vi "PT100.vi"(1 "R":dbl=-0.05) -> (0 "T":dbl)   [LabVIEW 2009]
panel:
  out "output cluster":cluster{dbl[], dbl[]}
  out "XY Graph":cluster{dbl[], dbl[]}(graph)
  in  "t":dbl=-0.05
  out "Rout":dbl
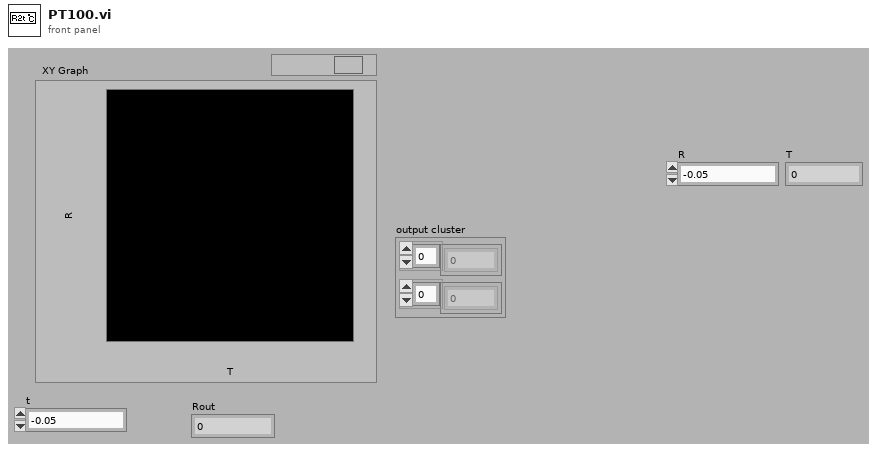
[diagram p1: front panel]
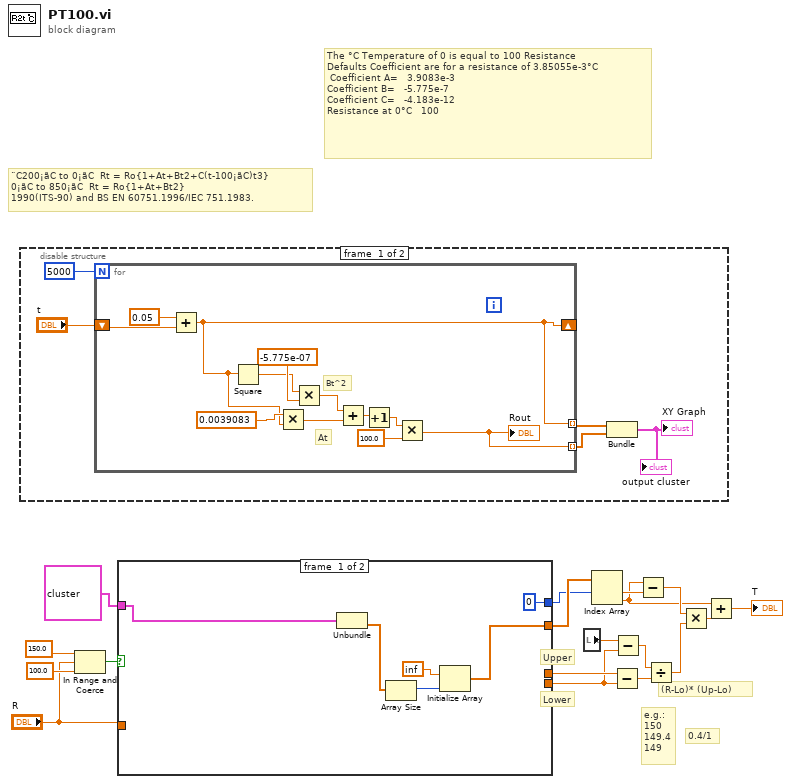
[diagram p0: block diagram]
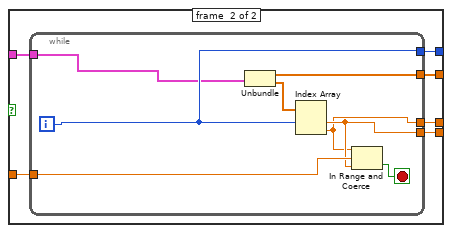
[diagram p3: hidden frame]
diagram:
  # "0.4/1"
  # "e.g.:\n150\n149.4\n149"
  # "(R-Lo)* (Up-Lo)"
  # "Lower"
  # "Upper"
  # "The °C Temperature of 0 is equal to 100 Resistance\nDefaults Coefficient are for a resistance of 3.85055e-3°C\n Coefficient A=   3.9083e-3 \nCoefficient B=   -5.775e-7 \nCoefficient C=   -4.183e-12 \nResistance at 0°C   100"
  # "¨C200¡ãC to 0¡ãC  Rt = Ro{1+At+Bt2+C(t-100¡ãC)t3} \n0¡ãC to 850¡ãC  Rt = Ro{1+At+Bt2} \n1990(ITS-90) and BS EN 60751.1996/IEC 751.1983."
  n1 = disable-structure shown="Enabled" {
    frame #0 {
      n2 = for {
        N: 5000 -> [_]
        shift-right: [w24] -> _
        shift-left: "t" -> [w26]
        tunnel: [w25] -> w20 mode=indexing
        tunnel: [w24] -> w21 mode=indexing
        # "At"
        # "Bt^2"
        n3 = Add(x=0.05, y=w26) -> (x+y=w24:dbl)
        n4 = Square(x=w24) -> (x^2=w34:dbl)
        n5 = Multiply(x=0.0039083 ("A"), y=w24) -> (x*y=w31:dbl)
        n6 = Multiply(x=w34, y=-5.775e-07 ("B")) -> (x*y=w32:dbl)
        n7 = Add(x=w32, y=w31) -> (x+y=w30:dbl)
        n8 = Increment(x=w30) -> (x+1=w29:dbl)
        n9 = Multiply(x=w29, y=100.0) -> (x*y=w25:dbl)
        "Rout" <- w25
      }
      n10 = Bundle(w21, w20) -> (→"XY Graph" →"output cluster":cluster{dbl[], dbl[]})  [unwired: 1 out]
    }
    frame #1 {
    }
  }
  n11 = In Range and Coerce(upper limit=150.0, x="R", lower limit=100.0) -> (In Range?=w17:bool)  [unwired: 1 out]
  n12 = case shown="True" w17 {
    tunnel: [w38 w47] -> w11
    tunnel: [_ w46] -> w16
    tunnel: [_ w45] -> w15
    tunnel: [0 w44] -> w10
    tunnel: "R" -> [_ w43]
    tunnel: cluster{dbl[], dbl[]} {array[5000 elements], array[5000 elements]} ("output cluster 2") -> [w41 w42]
    frame #0 {
      n13 = Unbundle(w41) -> (w36:dbl[])  [unwired: 1 out]
      n14 = Array Size(array=w36) -> (size(s)=w37:i32)
      n15 = Initialize Array(inf, w37) -> (w38:dbl[])
    }
    frame #1 {
      n16 = while {
        tunnel: [w53] -> w44
        tunnel: [w52] -> w47
        tunnel: w42 -> [w51]
        tunnel: [w48] -> w46
        tunnel: [w49] -> w45
        tunnel: w43 -> [w50]
        i -> [w53]
        stop <- w54 stop-if-true
        n17 = Unbundle(w51) -> (w52:dbl[], w55:dbl[])
        n18 = Index Array(array=w55, index #1=w53) -> (element #1=w49:dbl, element #2=w48:dbl)  [unwired: 1 in]
        n19 = In Range and Coerce(upper limit=w48, x=w50, lower limit=w49) -> (In Range?=w54:bool)  [unwired: 1 out]
      }
    }
  }
  n20 = local read "R"() -> (w14:dbl)
  n21 = Index Array(array=w11, index #1=w10) -> (element #1=w9:dbl, element #2=w5:dbl)  [unwired: 1 in]
  n22 = Subtract(x=w16, y=w15) -> (x-y=w13:dbl)
  n23 = Subtract(x=w14, y=w15) -> (x-y=w12:dbl)
  n24 = Subtract(x=w5, y=w9) -> (x-y=w8:dbl)
  n25 = Divide(x=w12, y=w13) -> (x/y=w7:dbl)
  n26 = Multiply(x=w8, y=w7) -> (x*y=w6:dbl)
  n27 = Add(x=w5, y=w6) -> (x+y=→"T":dbl)
